vi "Destroy.vi"(8 "error in":errorcluster, 11 "SignalGeneratorService in":refnum<class "ServiceBase.lvclass">) -> (0 "error out":errorcluster, 3 "SignalGeneratorService out":refnum<class "ServiceBase.lvclass">)   [LabVIEW 2019, in "gRPC-servicer.lvlib" / "ServiceBase.lvclass"]
uses:
  ServiceBase.lvclass
  ServiceBase.lvclass/ServiceBase.ctl
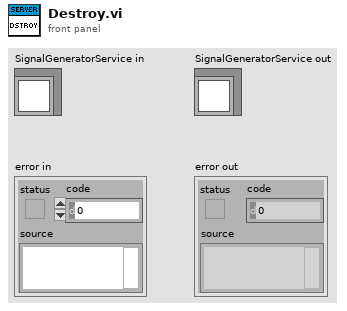
[diagram p1: front panel]
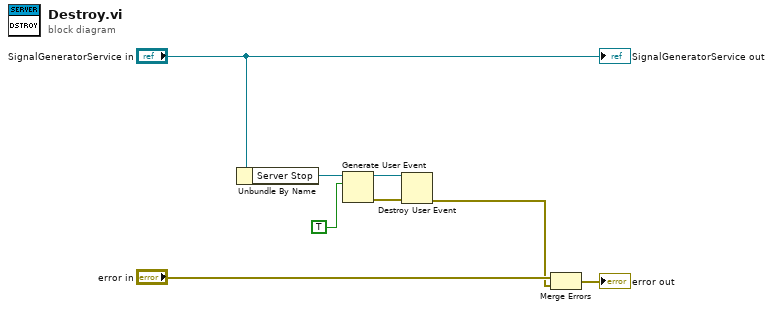
[diagram p0: block diagram]
diagram:
  n1 = Unbundle By Name("SignalGeneratorService in") -> ("Server Stop"=w3:refnum<user-event>)
  n2 = Generate User Event(user event=w3, event data cluster=TRUE) -> (user event out=w2:refnum<user-event>, error out=w7:errorcluster)  [unwired: 2 in]
  n3 = Destroy User Event(user event=w2, error in=w7) -> (error out=w5:errorcluster)
  n4 = Merge Errors("error in", w5) -> (→"error out":errorcluster)
  "SignalGeneratorService out" <- "SignalGeneratorService in"
